vi "PXI_MultiTrig.vi"() -> ()   [LabVIEW 2018, in "Visualization.lvlib" / "VisualizeSync.lvclass"]
doc: "This VI listens for any measurement data associated with the provided PluginName and displays it to the user for analysis. The display is only suitable for data coming from the RoomAlert Plugin."
uses:
  VisualizeSync.lvclass
  <vilib>/event_ctls.llb/usereventprio.ctl
  VisualizeBase/VisualizeBase_class/Requests/VisUserEventType.ctl
  <extravilib>/ChannelInstances/Tag-bool/Write With Abort.vi
  <extravilib>/ChannelInstances/Tag-bool/Read With Abort.vi
  <extravilib>/ChannelInstances/Tag-bool/Instantiate.vi
  <extravilib>/ChannelInstances/Tag-bool/EndpointRead.vi
  <vilib>/Utility/error.llb/Error Cluster From Error Code.vi
  <extravilib>/ChannelInstances/Tag-bool/Endpoint.vi
  <vilib>/ErrorRing/Error Ring.xnode
  <userlib>/NIST/NISTErrorLib/NISTErrorLib.lvlib
  VisualizeBase/VisualizeBase_class/VisualizeBase.lvclass
  <extravilib>/ChannelInstances/Tag-bool.lvlib
  TestClass/Test.lvclass
  Sync/SyncModule/SyncModule.lvlib
panel:
  in  "ModuleID":i32
  in  "Log Data":bool=TRUE
  in  "btnStop":bool
  in  "btnReset":bool
  in  "btnClearTest":bool
  out "LockStatus":bool
  out "Time Ref Offset (ns)":waveform(dbl)(graph)
  out "ErrorArray":errorcluster[](array[cluster])
  in  "PluginName":string="Sensor.RoomAlert1"
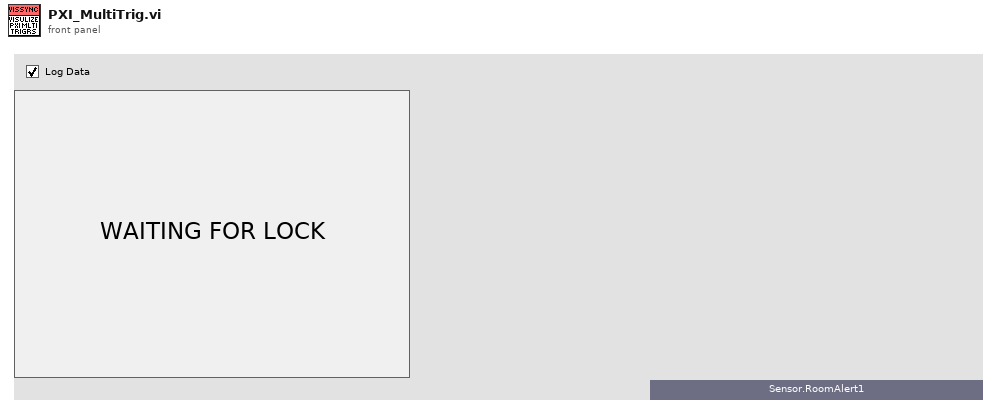
[diagram p1: front panel]
types:
  T1 = enum16{"open", "open or create", "create or replace", "create", "open (read-only)"}
  T2 = typedef "Visualization.lvlib/VisualizeBase.lvclass/VisRequestEvents.ctl" = cluster{"StopRequest":refnum<user-event>, "ResetRequest":refnum<user-event>, "FP Pop In or Out":refnum<user-event>}
  T3 = typedef "SyncModule.lvlib/SyncBroadcastEvents.ctl" = cluster{"DidInit":refnum<user-event>, "StatusUpdate":refnum<user-event>, "ErrorReport":refnum<user-event>, "DidStop":refnum<user-event>, "PathToINI":refnum<user-event>, "TriggerTime":refnum<user-event>, "LockStatus":refnum<user-event>, "Info":refnum<user-event>, "ClockProperties":refnum<user-event>, "SyncData":refnum<user-event>}
  T4 = cluster{"seconds since 1Jan1904":timestamp, "Time Ref Offset (ns)":dbl, "Lock":bool}
  T5 = typedef "Visualization.lvlib/VisualizeBase.lvclass/VisUserEventType.ctl" = cluster{"BusIndex":i8, "Data":variant}
  T6 = typedef "usereventprio.ctl" = enum32{"high priority", "normal priority"}
  T7 = typedef "Tag-bool.lvlib/))Channel.ctl" = refnum<queue>
  T8 = typedef "sizeaction.ctl" = enum32{"Minimized", "Maximized", "Resized"}
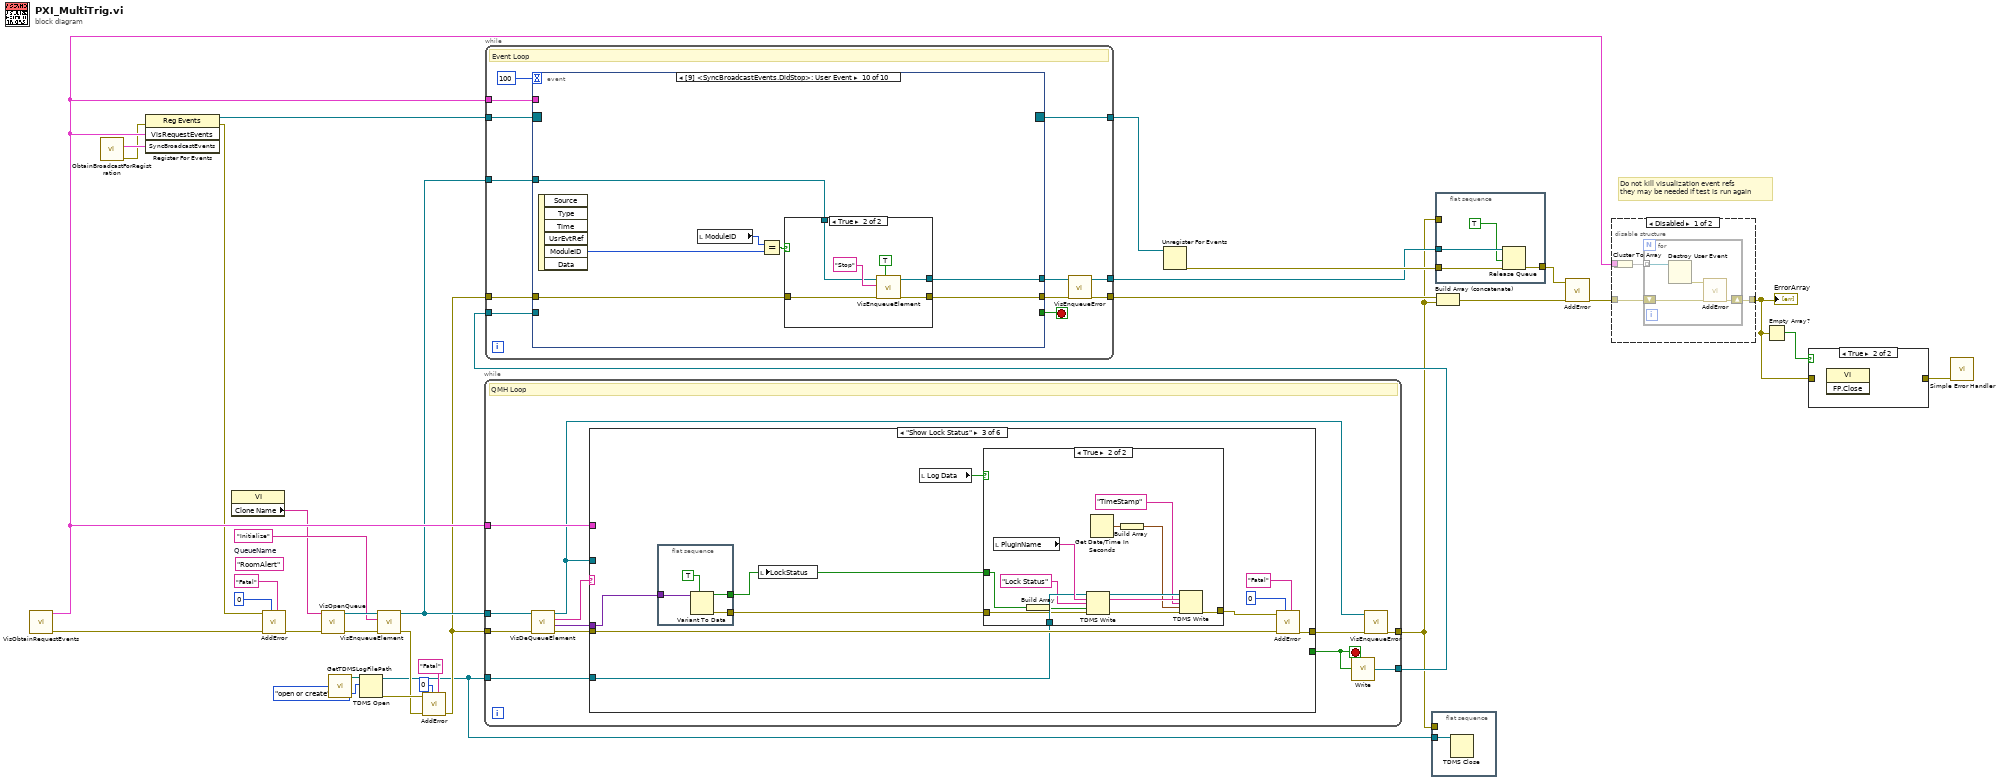
[diagram p0: block diagram]
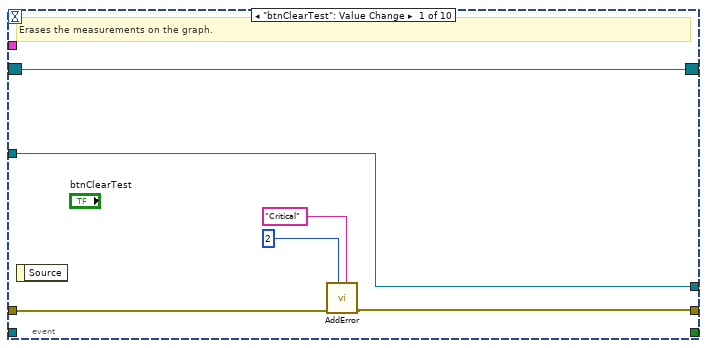
[diagram p3: hidden frame]
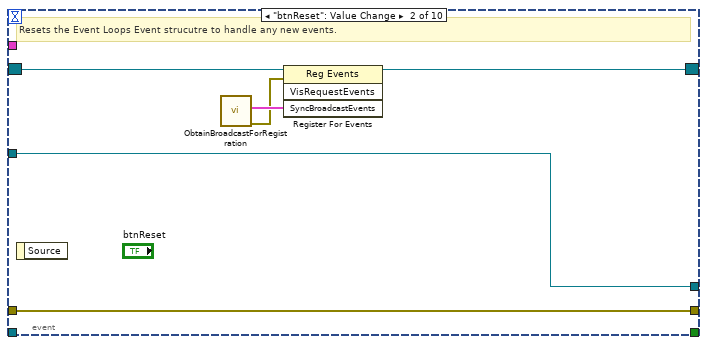
[diagram p4: hidden frame]
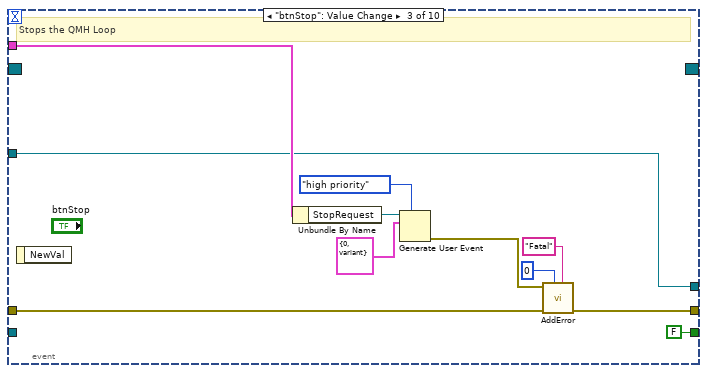
[diagram p5: hidden frame]
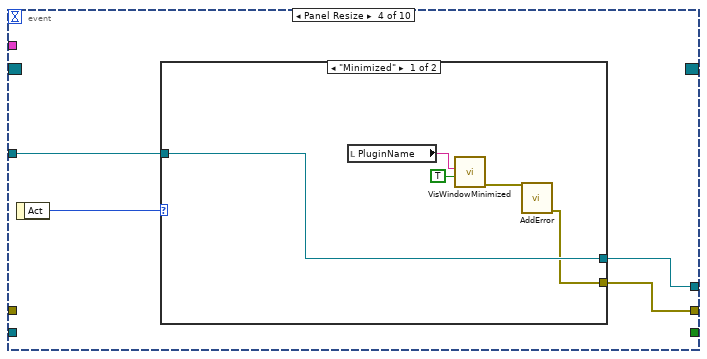
[diagram p6: hidden frame]
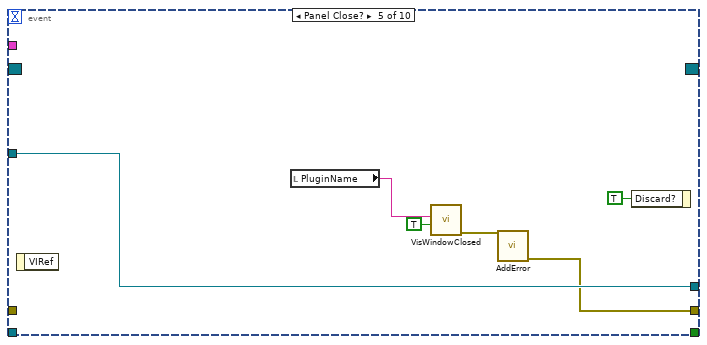
[diagram p8: hidden frame]
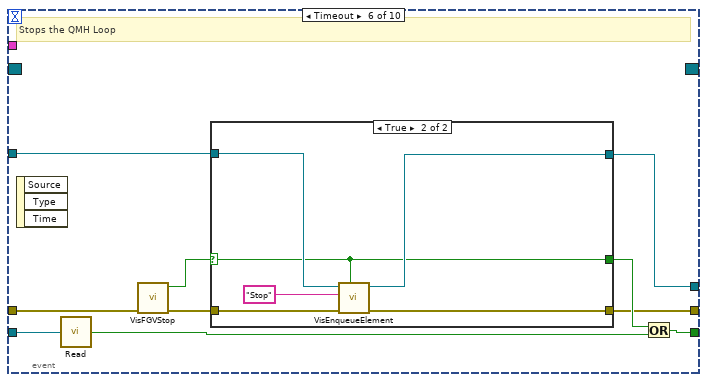
[diagram p9: hidden frame]
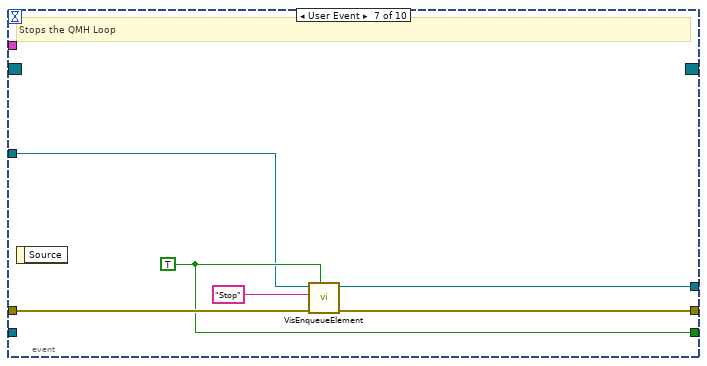
[diagram p11: hidden frame]
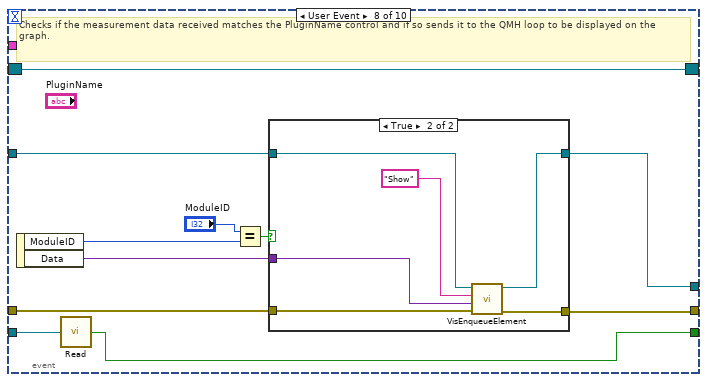
[diagram p12: hidden frame]
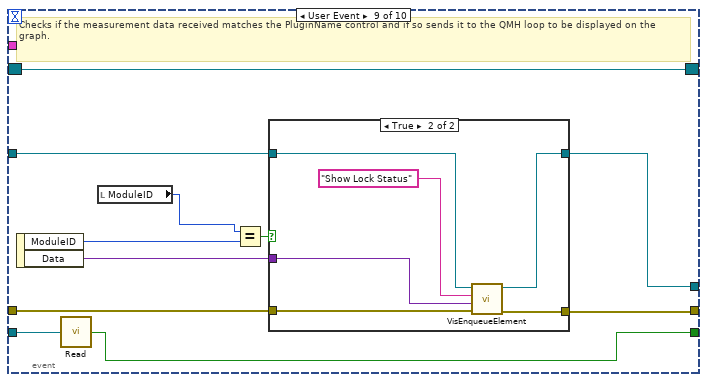
[diagram p14: hidden frame]
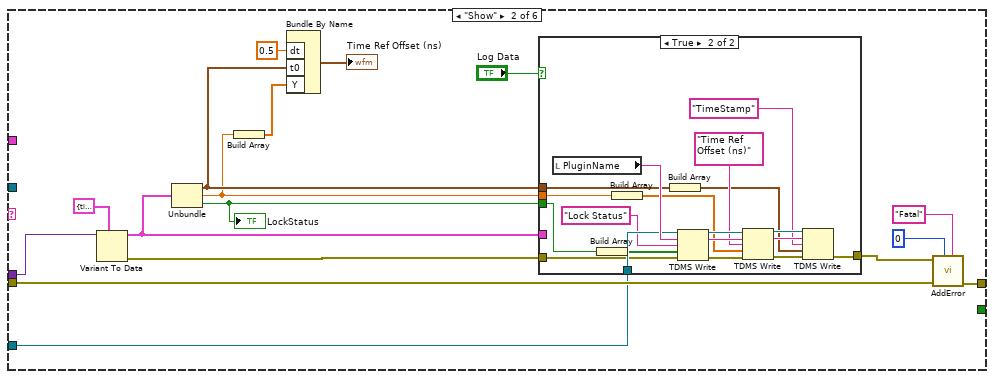
[diagram p18: hidden frame]
diagram:
  (unwired) "RoomAlert"  # QueueName
  # "Do not kill visualization event refs\nthey may be needed if test is run again"
  n1 = call "VisObtainRequestEvents.vi"() -> ("Error"=w25:errorcluster[], "VisRequestEvents"=w27:T2)  [unwired: 10 in]
  n2 = call "ObtainBroadcastForRegistration.vi"() -> ("error out"=w1:errorcluster, "SyncBroadcastEvents"=w2:T3)  [unwired: 10 in]
  n3 = register-events(error in=w1, w27, w2) -> (reference out=w34:refnum<event-registration>, error out=w24:errorcluster)  [unwired: 1 in]
  n4 = property class="VI"() -> ("Clone Name"=w12:string)  [unwired: 2 in, 2 out]
  n5 = call <userlib>:"AddError.vi"("Severity"="Fatal", "Priority"=u8 0, "ErrorArray In"=w25, "error in (no error)"=w24) -> ("ErrorArray Out"=w21:errorcluster[])  [unwired: 6 in, 1 out]
  n6 = call "VisOpenQueue.vi"("Error Array In"=w21, "QueueName"=w12) -> ("Error Array Out"=w19:errorcluster[], "queue out"=w20:refnum<queue>)  [unwired: 8 in]
  n7 = call "GetTDMSLogFilePath.vi"() -> ("TDMS Log File Path"=w11:path)  [unwired: 11 in]
  n8 = TDMS Open(10:T1."open or create" ("operation (0:open)"), 11:w11) -> (0:w8:errorcluster, 3:w4:refnum<k34>)  [unwired: 5 in]
  n9 = call "VisEnqueueElement.vi"("Error Array In"=w19, "Message"="Initialize", "queue in"=w20) -> ("Error Array Out"=w7:errorcluster[], "queue out"=w17:refnum<queue>)  [unwired: 7 in]
  n10 = call <userlib>:"AddError.vi"("Severity"="Fatal", "Priority"=u8 0, "ErrorArray In"=w7, "error in (no error)"=w8) -> ("ErrorArray Out"=w6:errorcluster[])  [unwired: 6 in, 1 out]
  n11 = while {
    tunnel: w6 -> [w40]
    tunnel: [w43] -> w3
    tunnel: w17 -> [w39]
    tunnel: w27 -> [w45]
    tunnel: [w36] -> w13
    tunnel: w4 -> [w35]
    stop <- w46 stop-if-true
    # "QMH Loop"
    n12 = call "VisDeQueueElement.vi"("Error Array In"=w40, "Queue In"=w39) -> ("Error Array Out"=w38:errorcluster[], "Data"=w41:variant, "Message"=w42:string, "Queue Out"=w37:refnum<queue>)  [unwired: 6 in]
    n13 = case shown="\"Show Lock Status\"" w42 {
      selector: w42 -> [_ _ _ w119 _ _]
      tunnel: w41 -> [_ w60 w90 _ w138 _]
      tunnel: w38 -> [w47 w63 w93 w117 _ w165]
      tunnel: [w47 w64 w94 w116 w128 w165] -> w44
      tunnel: [_ _ _ _ w134 TRUE] -> w46
      tunnel: w45 -> [_ _ _ _ w133 _]
      tunnel: w37 -> [_ _ _ _ w132 _]
      tunnel: w35 -> [_ w56 w87 _ _ _]
      frame "Initialize" {
      }
      frame "Show" {
        n14 = Variant To Data(type=T4 {"seconds since 1Jan1904"=timestamp(0 s since 1904-01-01), "Time Ref Offset (ns)"=0.0, "Lock"=FALSE} ("output cluster"), Variant=w60) -> (data=w54:T4, error out=w59:errorcluster)  [unwired: 1 in]
        n15 = Unbundle(w54) -> ("seconds since 1Jan1904"=w51:timestamp, "Time Ref Offset (ns)"=w49:dbl, "Lock"=w52:bool)
        "LockStatus" <- w52
        n16 = Build Array(w49) -> (w53:dbl[])
        n17 = Bundle By Name("dt"=0.5, "t0"=w51, "Y"=w53) -> (→"Time Ref Offset (ns)":waveform(dbl))  [unwired: 1 in]
        n18 = case shown="True" "Log Data" {
          tunnel: w59 -> [w65 w82]
          tunnel: [w65 w71] -> w58
          tunnel: w56 -> [_ w83]
          tunnel: w54 -> [_ _]
          tunnel: w52 -> [_ w80]
          tunnel: w49 -> [_ w75]
          tunnel: w51 -> [_ w68]
          frame False {
          }
          frame True {
            n19 = local read "PluginName"() -> (w84:string)
            n20 = Build Array(w80) -> (w81:bool[])
            n21 = Build Array(w75) -> (w66:dbl[])
            n22 = Build Array(w68) -> (w67:timestamp[])
            n23 = TDMS Write(0:w83, 5:w84, 7:"Lock Status" ("PluginName"), 9:w81, 11:w82) -> (4:w78:refnum<k34>, 6:w77:string, 15:w76:errorcluster)  [unwired: 1 in, 1 out]
            n24 = TDMS Write(0:w78, 5:w77, 7:"Time Ref Offset (ns)" ("PluginName"), 9:w66, 11:w76) -> (4:w74:refnum<k34>, 6:w73:string, 15:w72:errorcluster)  [unwired: 1 in, 1 out]
            n25 = TDMS Write(0:w74, 5:w73, 7:"TimeStamp" ("PluginName"), 9:w67, 11:w72) -> (15:w71:errorcluster)  [unwired: 1 in, 3 out]
          }
        }
        n26 = call <userlib>:"AddError.vi"("Severity"="Fatal" ("String"), "Priority"=u8 0, "ErrorArray In"=w63, "error in (no error)"=w58) -> ("ErrorArray Out"=w64:errorcluster[])  [unwired: 6 in, 1 out]
      }
      frame "Show Lock Status" {
        n27 = flat-sequence {
          tunnel: w90 -> [w98]
          tunnel: [w97] -> w89
          tunnel: [w95] -> w85
          frame #0 {
            n28 = Variant To Data(type=TRUE, Variant=w98) -> (data=w95:bool, error out=w97:errorcluster)  [unwired: 1 in]
          }
        }
        n29 = local write "LockStatus"(w85) -> ()
        n30 = local read "Log Data"() -> (w86:bool)
        n31 = case shown="True" w86 {
          tunnel: w89 -> [w99 w110]
          tunnel: [w99 w103] -> w88
          tunnel: w87 -> [_ w111]
          tunnel: w85 -> [_ w108]
          frame False {
          }
          frame True {
            n32 = local read "PluginName"() -> (w112:string)
            n33 = Build Array(w108) -> (w109:bool[])
            n34 = TDMS Write(0:w111, 5:w112, 7:"Lock Status" ("PluginName"), 9:w109, 11:w110) -> (4:w106:refnum<k34>, 6:w105:string, 15:w104:errorcluster)  [unwired: 1 in, 1 out]
            n35 = Get Date/Time In Seconds() -> (seconds since 1Jan1904=w100:timestamp)
            n36 = Build Array(w100) -> (w101:timestamp[])
            n37 = TDMS Write(0:w106, 5:w105, 7:"TimeStamp" ("PluginName"), 9:w101, 11:w104) -> (15:w103:errorcluster)  [unwired: 1 in, 3 out]
          }
        }
        n38 = call <userlib>:"AddError.vi"("Severity"="Fatal" ("String"), "Priority"=u8 0, "ErrorArray In"=w93, "error in (no error)"=w88) -> ("ErrorArray Out"=w94:errorcluster[])  [unwired: 6 in, 1 out]
      }
      frame Default {
        n39 = xnode "Error Ring"("parameter 0"=w119) -> ("error out"=w118:errorcluster)
        n40 = call <userlib>:"AddError.vi"("Severity"="Inform" ("String"), "Priority"=u8 5, "ErrorArray In"=w117, "error in (no error)"=w118) -> ("ErrorArray Out"=w116:errorcluster[], "error out"=w115:errorcluster)  [unwired: 6 in]
        n41 = call <vilib>:"Clear Errors.vi"("error in (no error)"=w115) -> ()  [unwired: 5 in, 2 out]
      }
      frame "Error" {
        n42 = Variant To Data(type=errorcluster[] [], Variant=w138) -> (data=w136:errorcluster[], error out=w127:errorcluster)  [unwired: 1 in]
        n43 = call <userlib>:"ParseErrors.vi"("ErrorArray"=w136) -> ("ErrorArray"=w135:errorcluster[])  [unwired: 8 in, 2 out]
        n44 = for {
          tunnel: w135 -> [w149] mode=indexing
          tunnel: [w143] -> w129 mode=concatenating
          tunnel: [w141] -> w134
          tunnel: w133 -> [w140]
          tunnel: w132 -> [w139]
          stop <- w141 stop-if-true
          n45 = call <userlib>:"GeneralHandler.vi"("error in (no error)"=w149) -> ("Severity"=w142:string, "Stop"=w146:bool, "Abort"=w147:bool, "Continue"=w148:bool)  [unwired: 6 in, 1 out]
          n46 = Build Array(w148, w147, w146) -> (w145:bool[])
          n47 = Boolean Array To Number(Boolean array=w145) -> (number=w144:u32)
          n48 = case shown="1" w144 {
            tunnel: [_ _ w154 w163] -> w143
            tunnel: w142 -> [_ _ _ w156]
            tunnel: [_ _ _ w158] -> w141
            tunnel: w140 -> [_ _ _ w157]
            tunnel: w139 -> [_ _ w150 _]
            frame 0, Default {
              # "No Dialog"
            }
            frame 1 {
              # "Continue"
            }
            frame 2 {
              # "Abort, Flush Queue"
              n49 = Flush Queue(queue=w150) -> (error out=w153:errorcluster)  [unwired: 1 in, 2 out]
              n50 = call <userlib>:"AddError.vi"("Severity"="Critical" ("String"), "Priority"=u8 1, "error in (no error)"=w153) -> ("ErrorArray Out"=w154:errorcluster[])  [unwired: 7 in, 1 out]
            }
            frame 4 {
              # "Stop"
              n51 = Unbundle By Name(w157) -> ("StopRequest"=w164:refnum<user-event>)
              n52 = Equal?(x=w156, y="Fatal" ("x")) -> (x = y?=w158:bool)
              n53 = Generate User Event(priority (normal)=usereventprio."high priority", user event=w164, event data cluster=T5 {"BusIndex"=0, "Data"=variant} ("event data")) -> (error out=w162:errorcluster)  [unwired: 1 in, 1 out]
              n54 = call <userlib>:"AddError.vi"("error in (no error)"=w162) -> ("ErrorArray Out"=w163:errorcluster[], "error out"=w159:errorcluster)  [unwired: 9 in]
              n55 = call <vilib>:"Clear Errors.vi"("error in (no error)"=w159) -> ()  [unwired: 5 in, 2 out]
            }
          }
        }
        n56 = call <userlib>:"AddError.vi"("Severity"="Critical", "Priority"=u8 2, "ErrorArray In"=w129, "error in (no error)"=w127) -> ("ErrorArray Out"=w128:errorcluster[])  [unwired: 6 in, 1 out]
      }
      frame "Stop" {
      }
    }
    n57 = call <extravilib>:"Write.vi"("element"=w46) -> ("channel"=w36:T7)  [unwired: 1 out]
    n58 = call "VisEnqueueError.vi"("Error Array In"=w44, "Queue in"=w37) -> ("Error Array Out"=w43:errorcluster[])  [unwired: 8 in, 1 out]
  }
  n59 = while {
    tunnel: w34 -> [w178]
    tunnel: [w172] -> w32
    tunnel: [w176] -> w33
    tunnel: w27 -> [w175]
    tunnel: w6 -> [w174]
    tunnel: w17 -> [w173]
    tunnel: [w169] -> w16
    tunnel: w13 -> [w167]
    stop <- w177 stop-if-true
    # "Event Loop"
    n60 = event shown="[9] <SyncBroadcastEvents.DidStop>: User Event" {
      selector: w178 -> [w180 w190 _ _ _ _ _ w249 w268 _]
      dyn-events: [w180 w189 _ _ _ _ _ w249 w268 _] -> w176
      timeout: 100 -> [_ _ _ _ _ _ _ _ _ _]
      tunnel: [_ _ FALSE ("Priority? (F)") _ _ w218 w239 w246 w265 _] -> w177
      tunnel: [w181 w188 w194 w204 w212 w220 w241 w251 w270 w285] -> w171
      tunnel: w175 -> [_ _ w193 _ _ _ _ _ _ _]
      tunnel: w174 -> [w182 w188 w201 _ _ w223 w242 w252 w271 w284]
      tunnel: w173 -> [w179 w187 w191 w203 w216 w222 w237 w253 w272 w283]
      tunnel: [w179 w187 w191 w202 w216 w221 w240 w250 w269 w286] -> w170
      tunnel: w167 -> [_ _ _ _ _ w227 _ w247 w266 _]
      event "btnClearTest": Value Change {
        # "Erases the measurements on the graph."
        n61 = event-data() -> ()  [unwired: 1 in, 1 out]
        n62 = call <userlib>:"AddError.vi"("Severity"="Critical", "Priority"=u8 2, "ErrorArray In"=w182) -> ("ErrorArray Out"=w181:errorcluster[])  [unwired: 7 in, 1 out]
      }
      event "btnReset": Value Change {
        # "Resets the Event Loops Event strucutre to handle any new events."
        n63 = event-data() -> ()  [unwired: 1 in, 1 out]
        n64 = call "ObtainBroadcastForRegistration.vi"() -> ("error out"=w185:errorcluster, "SyncBroadcastEvents"=w186:T3)  [unwired: 10 in]
        n65 = register-events(reference=w190, error in=w185, w186) -> (reference out=w189:refnum<event-registration>)  [unwired: 1 in, 1 out]
      }
      event "btnStop": Value Change {
        # "Stops the QMH Loop"
        n66 = event-data() -> ()  [unwired: 1 in, 1 out]
        n67 = Unbundle By Name(w193) -> ("StopRequest"=w199:refnum<user-event>)
        n68 = Generate User Event(priority (normal)=usereventprio."high priority", user event=w199, event data cluster=T5 {"BusIndex"=0, "Data"=variant} ("event data")) -> (error out=w200:errorcluster)  [unwired: 1 in, 1 out]
        n69 = call <userlib>:"AddError.vi"("Severity"="Fatal" ("String"), "Priority"=u8 0, "ErrorArray In"=w201, "error in (no error)"=w200) -> ("ErrorArray Out"=w194:errorcluster[])  [unwired: 6 in, 1 out]
      }
      event Panel Resize {
        n70 = event-data() -> ("Act"=w205:T8)  [unwired: 1 in]
        n71 = case shown="\"Minimized\"" w205 {
          tunnel: [w207 _] -> w204
          tunnel: w203 -> [w208 w211]
          tunnel: [w208 w211] -> w202
          frame "Minimized" {
            n72 = local read "PluginName"() -> (w210:string)
            n73 = call "VisWindowMinimized.vi"("Window Minimized?"=TRUE ("Window Minimized or Clozed?"), "Module Name"=w210) -> ("error out"=w209:errorcluster)  [unwired: 9 in]
            n74 = call <userlib>:"AddError.vi"("error in (no error)"=w209) -> ("ErrorArray Out"=w207:errorcluster[])  [unwired: 9 in, 1 out]
          }
          frame "Maximized", Default {
          }
        }
      }
      event Panel Close? {
        n75 = event-data() -> ()  [unwired: 1 in, 1 out]
        n76 = local read "PluginName"() -> (w215:string)
        n77 = call "VisWindowClosed.vi"("Window Closed?"=TRUE ("Window Minimized or Clozed?"), "Module Name"=w215) -> ("error out"=w214:errorcluster)  [unwired: 9 in]
        n78 = call <userlib>:"AddError.vi"("error in (no error)"=w214) -> ("ErrorArray Out"=w212:errorcluster[])  [unwired: 9 in, 1 out]
        n79 = event-data("Discard?"=TRUE) -> ()  [unwired: 1 in, 1 out]
      }
      event Timeout {
        # "Stops the QMH Loop"
        n80 = event-data() -> ()  [unwired: 1 in, 3 out]
        n81 = call <extravilib>:"Read.vi"("channel"=w227) -> ("element"=w219:bool)  [unwired: 1 in, 1 out]
        n82 = call "VisFGVStop.vi"("Error In"=w223) -> ("Error Out"=w225:errorcluster[], "Value"=w226:bool)  [unwired: 9 in]
        n83 = case shown="True" w226 {
          selector: w226 -> [w228 w231]
          tunnel: [w230 w234] -> w220
          tunnel: w225 -> [w230 w235]
          tunnel: w222 -> [w229 w233]
          tunnel: [w229 w232] -> w221
          tunnel: [w228 w231] -> w224
          frame False {
          }
          frame True {
            n84 = call "VisEnqueueElement.vi"("Priority? (F)"=w231, "Error Array In"=w235, "Message"="Stop", "queue in"=w233) -> ("Error Array Out"=w234:errorcluster[], "queue out"=w232:refnum<queue>)  [unwired: 6 in]
          }
        }
        n85 = Or(x=w224, y=w219) -> (x .or. y?=w218:bool)
      }
      event User Event {
        w239 = TRUE ("Priority? (F)")
        # "Stops the QMH Loop"
        n86 = event-data() -> ()  [unwired: 1 in, 1 out]
        n87 = call "VisEnqueueElement.vi"("Priority? (F)"=w239, "Error Array In"=w242, "Message"="Stop", "queue in"=w237) -> ("Error Array Out"=w241:errorcluster[], "queue out"=w240:refnum<queue>)  [unwired: 6 in]
      }
      event User Event {
        # "Checks if the measurement data received matches the PluginName control and if so sends it to the QMH loop to be displayed on the graph."
        n88 = event-data() -> ("ModuleID"=w244:i32, "Data"=w245:variant)  [unwired: 1 in]
        n89 = call <extravilib>:"Read.vi"("channel"=w247) -> ("element"=w246:bool)  [unwired: 1 in, 1 out]
        n90 = Equal?(x="ModuleID", y=w244) -> (x = y?=w248:bool)
        n91 = case shown="True" w248 {
          tunnel: [w254 w260] -> w251
          tunnel: w253 -> [w255 w259]
          tunnel: w252 -> [w254 w261]
          tunnel: [w255 w258] -> w250
          tunnel: w245 -> [_ w256]
          frame False {
          }
          frame True {
            n92 = call "VisEnqueueElement.vi"("Error Array In"=w261, "Data"=w256, "Message"="Show", "queue in"=w259) -> ("Error Array Out"=w260:errorcluster[], "queue out"=w258:refnum<queue>)  [unwired: 6 in]
          }
        }
      }
      event User Event {
        # "Checks if the measurement data received matches the PluginName control and if so sends it to the QMH loop to be displayed on the graph."
        n93 = event-data() -> ("ModuleID"=w263:i32, "Data"=w264:variant)  [unwired: 1 in]
        n94 = call <extravilib>:"Read.vi"("channel"=w266) -> ("element"=w265:bool)  [unwired: 1 in, 1 out]
        n95 = local read "ModuleID"() -> (w262:i32)
        n96 = Equal?(x=w262, y=w263) -> (x = y?=w267:bool)
        n97 = case shown="True" w267 {
          tunnel: [w273 w279] -> w270
          tunnel: w272 -> [w274 w278]
          tunnel: w271 -> [w273 w280]
          tunnel: [w274 w277] -> w269
          tunnel: w264 -> [_ w275]
          frame False {
          }
          frame True {
            n98 = call "VisEnqueueElement.vi"("Error Array In"=w280, "Data"=w275, "Message"="Show Lock Status", "queue in"=w278) -> ("Error Array Out"=w279:errorcluster[], "queue out"=w277:refnum<queue>)  [unwired: 6 in]
          }
        }
      }
      event User Event {
        n99 = event-data() -> ("ModuleID"=w281:i32)  [unwired: 1 in, 5 out]
        n100 = local read "ModuleID"() -> (w282:i32)
        n101 = Equal?(x=w282, y=w281) -> (x = y?=w287:bool)
        n102 = case shown="True" w287 {
          tunnel: [w288 w293] -> w285
          tunnel: [w289 w292] -> w286
          tunnel: w283 -> [w289 w291]
          tunnel: w284 -> [w288 w290]
          frame False {
          }
          frame True {
            n103 = call "VisEnqueueElement.vi"("Priority? (F)"=TRUE, "Error Array In"=w290, "Message"="Stop", "queue in"=w291) -> ("Error Array Out"=w293:errorcluster[], "queue out"=w292:refnum<queue>)  [unwired: 6 in]
          }
        }
      }
    }
    n104 = call "VisEnqueueError.vi"("Error Array In"=w171, "Queue in"=w170) -> ("Error Array Out"=w172:errorcluster[], "Queue out"=w169:refnum<queue>)  [unwired: 8 in]
  }
  n105 = Unregister For Events(event registration refnum=w33) -> (error out=w31:errorcluster)  [unwired: 1 in]
  n106 = flat-sequence {
    tunnel: w4 -> [w296]
    tunnel: w3 -> [_]
    frame #0 {
      n107 = TDMS Close(11:w296) -> ()  [unwired: 1 in, 2 out]
    }
  }
  n108 = flat-sequence {
    tunnel: w31 -> [w300]
    tunnel: [w299] -> w29
    tunnel: w16 -> [w298]
    tunnel: w3 -> [_]
    frame #0 {
      n109 = Release Queue(queue=w298, force destroy? (F)=TRUE, error in (no error)=w300) -> (error out=w299:errorcluster)  [unwired: 2 out]
    }
  }
  n110 = Build Array (concatenate)(w32, w3) -> (w30:errorcluster[])
  n111 = call <userlib>:"AddError.vi"("ErrorArray In"=w30, "error in (no error)"=w29) -> ("ErrorArray Out"=w28:errorcluster[])  [unwired: 8 in, 1 out]
  n112 = disable-structure shown="Disabled" {
    disable-tunnel: w28 -> [w303 w309]
    disable-tunnel: w27 -> [w302 _]
    disable-tunnel: [w301 w309] -> w15
    frame Disabled {
      n113 = Cluster To Array(cluster=w302) -> (array=w304:refnum<user-event>[])
      n114 = for {
        tunnel: w304 -> [w308] mode=indexing
        shift-right: [w307] -> w301
        shift-left: w303 -> [w306]
        n115 = Destroy User Event(user event=w308) -> (error out=w305:errorcluster)  [unwired: 1 in]
        n116 = call <userlib>:"AddError.vi"("ErrorArray In"=w306, "error in (no error)"=w305) -> ("ErrorArray Out"=w307:errorcluster[])  [unwired: 8 in, 1 out]
      }
    }
    frame Enabled {
    }
  }
  "ErrorArray" <- w15
  n117 = Empty Array?(array=w15) -> (empty?=w26:bool)
  n118 = case shown="True" w26 {
    tunnel: [w310 _] -> w14
    tunnel: w15 -> [w311 _]
    frame False {
      n119 = Merge Errors(w311) -> (w310:errorcluster)
    }
    frame True {
      n120 = invoke class="VI" method="FP.Close"() -> ()  [unwired: 3 in, 3 out]
    }
  }
  n121 = call <vilib>:"Simple Error Handler.vi"("error in (no error)"=w14) -> ()  [unwired: 4 in, 5 out]
